vi "vector_to_xy.vi"(8 "threshold":dbl=10.0, 9 "Max Speed":dbl=3.0, 11 "Initial X, Y, BEARING":cluster{dbl, dbl, dbl}) -> (3 "Final X, Y, BEARING":cluster{dbl, dbl, dbl}={-4.992843950545212, 691.6700659397637, 27.314769230769336})   [LabVIEW 2017]
uses:
  040-typeDefs/Position.ctl
  <vilib>/myRIO/Common/Instrument Driver Framework/myRIO v1.0/Encoder/typedefs/Encoder Signal Mode.ctl
  <vilib>/myRIO/Instrument Drivers/Onboard IO/Encoder/typedefs/Encoder Reference.ctl
  <vilib>/myRIO/Common/Instrument Driver Framework/Utilities/typedefs/myRIO Generic Hardware Reference.ctl
  <vilib>/myRIO/Common/Instrument Driver Framework/Utilities/typedefs/Hardware Version Enum.ctl
  <vilib>/myRIO/Common/Instrument Driver Framework/Utilities/typedefs/myRIO v1.0 Reference.ctl
  <vilib>/myRIO/Common/Instrument Driver Framework/Utilities/typedefs/Generic FPGA Reference.ctl
  <vilib>/myRIO/Common/Instrument Driver Framework/myRIO v1.0/Encoder/typedefs/Encoder Channels Enum.ctl
  <vilib>/myRIO/Common/Instrument Driver Framework/myRIO v1.0/Encoder/typedefs/Encoder Configuration v1.0.ctl
  <vilib>/userdefined/High Color/nirio_resource_hc.ctl
  <vilib>/myRIO/Common/Instrument Driver Framework/Utilities/vis/Is FPGA Ref Available.vi
  <vilib>/myRIO/Common/Instrument Driver Framework/myRIO v1.0/Encoder/vis/myRIO v1.1 Open Encoder.vi
  <vilib>/myRIO/Instrument Drivers/Onboard IO/Encoder/vis/Read.vi
  <vilib>/myRIO/Common/Instrument Driver Framework/Utilities/vis/Validate Channels.vi
  <vilib>/myRIO/Common/Instrument Driver Framework/myRIO v1.0/Encoder/vis/myRIO v1.0 Reserve Encoder.vi
  <vilib>/myRIO/Common/Instrument Driver Framework/myRIO v1.0/Encoder/vis/myRIO v1.0 Build MUX Configuration Encoder.vi
  <vilib>/myRIO/Common/Instrument Driver Framework/myRIO v1.0/Resource Manager/vis/myRIO v1.0 Reserve Channel List.vi
  <vilib>/myRIO/Common/Instrument Driver Framework/myRIO v1.0/Resource Manager/vis/myRIO v1.0 Create Configuration List.vi
  <vilib>/myRIO/Common/Instrument Driver Framework/myRIO v1.0/Resource Manager/vis/myRIO v1.0 Reserve Channel.vi
  <vilib>/myRIO/Common/Instrument Driver Framework/myRIO v1.0/Resource Manager/vis/myRIO v1.0 Unreserve Channel.vi
  <vilib>/myRIO/Common/Instrument Driver Framework/myRIO v1.0/Resource Manager/vis/myRIO v1.0 Build Mutex Name.vi
  <vilib>/Utility/VariantDataType/GetNumericInfo.vi
  <vilib>/Utility/error.llb/Error Cluster From Error Code.vi
  <vilib>/myRIO/Common/Instrument Driver Framework/myRIO v1.0/myRIO v1.1 Open.vi
  <vilib>/myRIO/Common/Instrument Driver Framework/Utilities/vis/IO Manager.vi
  <vilib>/myRIO/Common/Instrument Driver Framework/Utilities/vis/Configuration Manager.vi
  <vilib>/myRIO/Common/Instrument Driver Framework/myRIO v1.0/Resource Manager/vis/myRIO v1.0 Configure IO.vi
  <vilib>/myRIO/Common/Instrument Driver Framework/myRIO v1.0/myRIO v1.0 Close.vi
  <vilib>/myRIO/Common/Instrument Driver Framework/myRIO v1.0/Encoder/vis/myRIO v1.0 Configure Encoder.vi
  <vilib>/myRIO/Common/Instrument Driver Framework/myRIO v1.0/Encoder/vis/myRIO v1.0 Read Encoder.vi
  <vilib>/addons/control/pid/pid.llb/PID (DBL).vi
  <vilib>/myRIO/Express VI/Onboard IO/Encoder/Encoder Express VI.xnode
  <vilib>/myRIO/Instrument Drivers/Onboard IO/Encoder/vis/myRIO Encoder Open.xnode
  <vilib>/myRIO/Common/Instrument Driver Framework/myRIO v1.0/Encoder/typedefs/Encoder Count Direction Enum.ctl
  <vilib>/addons/control/pid/NI_PID_pid.lvlib
  <vilib>/myRIO/Instrument Drivers/Onboard IO/Encoder/Encoder.lvlib
panel:
  out "X, Y, BEARING 2":cluster{dbl, dbl, dbl}={-5.221699480492852, 691.22694677004, 27.197538461538567}
  in  "Array":T1[](array[typedef])=[{"X Pos"=100.0, "Y Pos"=150.0, "Bearing"=0.0}, {"X Pos"=-100.0, "Y Pos"=300.0, "Bearing"=0.0}, {"X Pos"=100.0, "Y Pos"=450.0, "Bearing"=0.0}, {"X Pos"=0.0, "Y Pos"=600.0, "Bearing"=0.0}, {"X Pos"=0.0, "Y Pos"=700.0, "Bearing"=0.0}]
  in  "Min Speed":dbl=1.0
  out "PID Angle":cluster{"Bearing":dbl, dbl}(graph)={"Bearing"=30.937872520261912, 27.314769230769336}
  out "XY Graph":cluster{"X":dbl, "Y":dbl}[](graph)=[{"X"=-5.221699480492852, "Y"=691.22694677004}, {"X"=-4.992843950545212, "Y"=691.6700659397637}]
  in  "PID gains":T2={"proportional gain (Kc)"=0.05, "integral time (Ti, min)"=0.05, "derivative time (Td, min)"=0.0} {"derivative time (Td, min)" format="%.3f"; "integral time (Ti, min)" format="%.3f"; "proportional gain (Kc)" format="%.3f"}
  in  "stop":bool
  out "OUTPUT B":dbl(slide)=0.6 scale=-10.0..10.0
  out "OUTPUT A":dbl(slide)=1.4816000000000713 scale=-10.0..10.0
  out "PID A":T3(graph)={"Setpoint"=1.3414004312104115, "output"=0.09438687184526344, "dx/dt"=1.4816000000000713}
  out "PID B":T3(graph)={"Setpoint"=0.6585995687895885, "output"=0.05545907338162134, "dx/dt"=0.6}
  out "Setpoint A":dbl(slide)=1.3414004312104115 scale=-10.0..10.0
  out "Setpoint B":dbl(slide)=0.6585995687895885 scale=-10.0..10.0
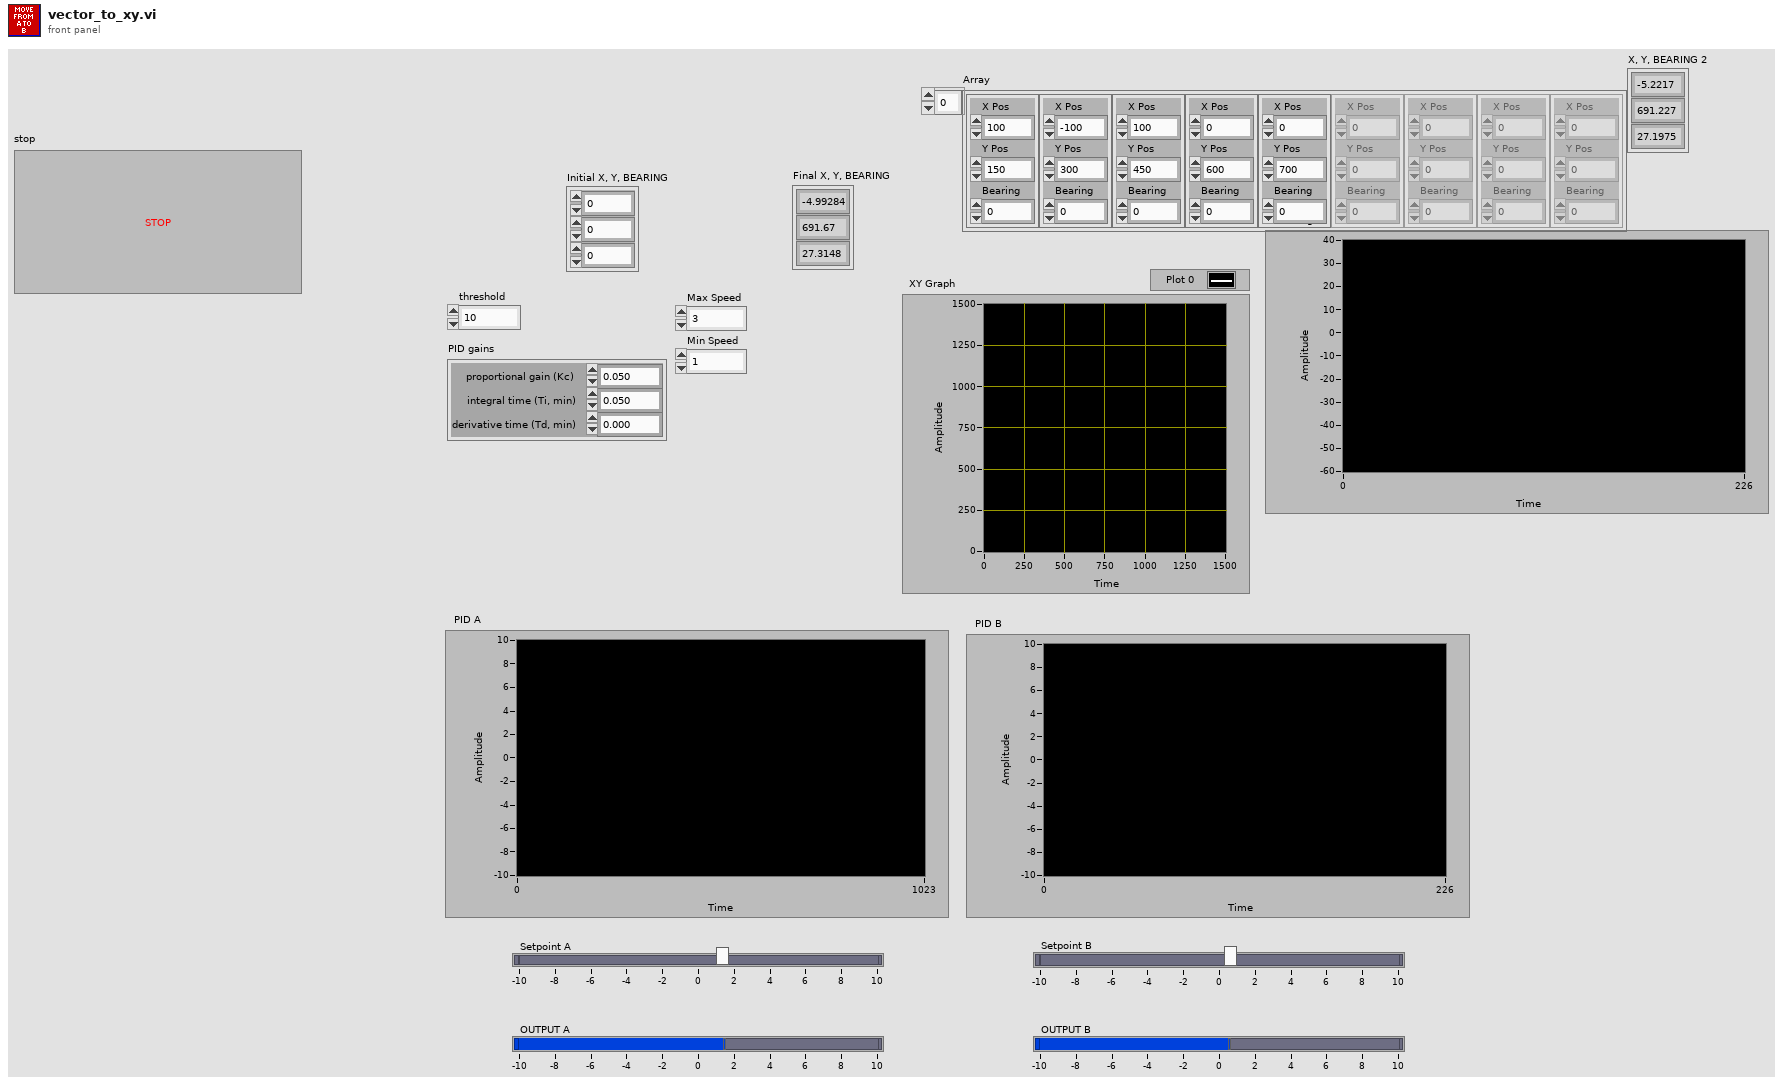
[diagram p1: front panel]
types:
  T1 = typedef "Position.ctl" = cluster{"X Pos":dbl, "Y Pos":dbl, "Bearing":dbl}
  T2 = cluster{"proportional gain (Kc)":dbl, "integral time (Ti, min)":dbl, "derivative time (Td, min)":dbl}
  T3 = cluster{"Setpoint":dbl, "output":dbl, "dx/dt":dbl}
  T4 = typedef "Encoder.lvlib/Encoder Reference.ctl" = cluster{"myRIO Reference":T5, "Encoder Channels Enum":T9}
  T5 = typedef "myRIO Generic Hardware Reference.ctl" = cluster{"myRIO Model":T6, "myRIO Hardware Reference":T7}
  T6 = typedef "Hardware Version Enum.ctl" = enum16{"Unknown", "myRIO-1900", "myRIO-1950", "roboRIO", "NI ELVIS RIO CM"}
  T7 = typedef "myRIO v1.0 Reference.ctl" = cluster{"Generic FPGA Reference":T8, "Allow multiple opens":bool}
  T8 = typedef "Generic FPGA Reference.ctl" = refnum<k20>
  T9 = typedef "Encoder Channels Enum.ctl" = enum16{"Not Connected", "C/ENC0", "C/ENC1", "A/ENC", "B/ENC", "DIO/ENC0", "DIO/ENC1", "DIO/ENC2", "DIO/ENC3", "DIO/ENC4"}
  T10 = typedef "Encoder Signal Mode.ctl" = enum16{"Quadrature phase signal", "Step and direction signal"}
  T11 = typedef "nirio_resource_hc.ctl" = tag
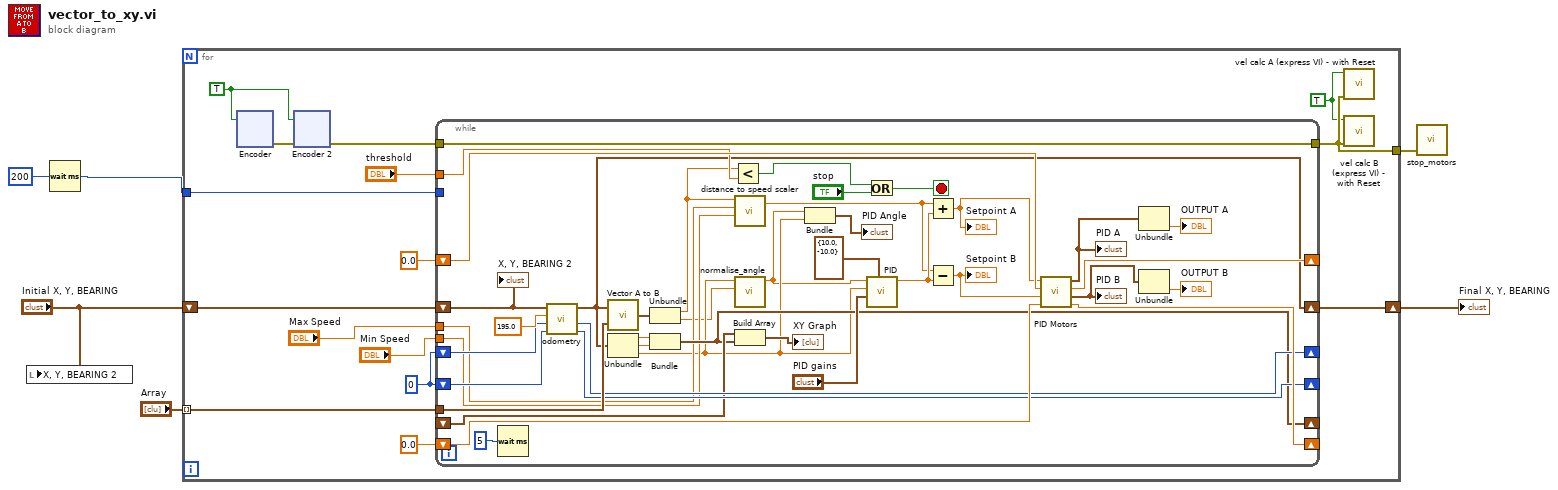
[diagram p0: block diagram]
diagram:
  n1 = local write "X, Y, BEARING 2"("Initial X, Y, BEARING") -> ()
  n2 = Wait (ms)(milliseconds to wait=u32 200) -> (millisecond timer value=w1:u32)
  n3 = for {
    shift-right: [w15] -> w6
    shift-left: "Initial X, Y, BEARING" -> [w14]
    tunnel: "Array" -> [w13] mode=indexing
    tunnel: [w9] -> w4
    tunnel: w1 -> [w7]
    w8 = TRUE ("Reinitialise")
    w11 = TRUE
    w18 = 0 ("ENCA OUT")
    n4 = xnode "Encoder"("Reset Counter"=w11) -> ("error out"=w12:errorcluster)  [unwired: 1 in, 3 out]
    n5 = xnode "Encoder 2"("error in (no error)"=w12, "Reset Counter"=w11) -> ("error out"=w10:errorcluster)  [unwired: 3 out]
    n6 = while {
      tunnel: w10 -> [w148]
      shift-right: [w150] -> _
      shift-left: 0.0 ("output A") -> [w151]
      shift-right: [w153] -> _
      shift-left: 0.0 ("output B") -> [w152]
      tunnel: [w148] -> w9
      tunnel: w13 -> [w139]
      tunnel: "threshold" -> [w135]
      shift-right: [w131] -> _
      shift-left: w18 -> [w133]
      shift-right: [w130] -> _
      shift-left: w18 -> [w132]
      shift-right: [w128] -> w15
      shift-left: w14 -> [w129]
      shift-right: [w124] -> _
      shift-left: _ -> [w125]
      tunnel: "Max Speed" -> [w119]
      tunnel: "Min Speed" -> [w118]
      tunnel: w7 -> [_]
      stop <- w136 stop-if-true
      n7 = Wait (ms)(milliseconds to wait=5 ("ENCB OUT")) -> ()  [unwired: 1 out]
      n8 = call "odometry.vi"("ENCB in"=w132, "ENCA in"=w133, "wheelbase"=195.0, "Position"=w129) -> ("ENCB OUT"=w130:i32, "ENCA OUT"=w131:i32, "X, Y, BEARING"=w128:cluster{dbl, dbl, dbl})  [unwired: 4 in]
      n9 = call "Vector A to B.vi"("Destination"=w139, "Current"=w128) -> ("vector"=w138:cluster{dbl, "Bearing":dbl})
      n10 = Unbundle(w128) -> (w126:dbl, w127:dbl, w116:dbl)
      n11 = Unbundle(w138) -> (w120:dbl, "Bearing"=w115:dbl)
      n12 = Bundle(w126, w127) -> (w124:cluster{dbl, dbl})  [unwired: 1 in]
      n13 = Less?(x=w120, y=w135) -> (x < y?=w134:bool)
      n14 = call "distance to speed scaler.vi"("Min Speed"=w118, "Max Speed"=w119, "Distance (mm)"=w120) -> ("Speed (0..10)"=w121:dbl)  [unwired: 2 in]
      n15 = call "normalise_angle.vi"("target -180 .. 180"=w115, "current"=w116) -> ("travel_direction"=w114:dbl)  [unwired: 9 in]
      n16 = Build Array(w125, w124) -> (→"XY Graph":cluster{dbl, dbl}[])
      n17 = Bundle("travel_direction"=w114, w116) -> (→"PID Angle":cluster{"travel_direction":dbl, dbl})  [unwired: 1 in]
      n18 = Or(x=w134, y="stop") -> (x .or. y?=w136:bool)
      n19 = call-poly <vilib>:"PID.vi"("output range"=cluster{"output high":dbl, "output low":dbl} {"output high"=10.0, "output low"=-10.0}, "PID gains"="PID gains", "process variable"=w116, "setpoint"=w114) -> ("output"=w143:dbl)  [unwired: 6 in, 1 out]
      n20 = Add(x=w121, y=w143) -> (x+y=w140:dbl)
      "Setpoint A" <- w140
      n21 = Subtract(x=w121, y=w143) -> (x-y=w141:dbl)
      "Setpoint B" <- w141
      n22 = call "PID Motors.vi"("input B"=w152, "Speed B"=w141, "input A"=w151, "Speed A"=w140) -> ("output B"=w153:dbl, "Speed B0"=w146:T3, "output A"=w150:dbl, "Speed A0"=w147:T3)
      "PID B" <- w146
      "PID A" <- w147
      n23 = Unbundle(w147) -> ("dx/dt"=→"OUTPUT A":dbl)  [unwired: 2 out]
      n24 = Unbundle(w146) -> ("dx/dt"=→"OUTPUT B":dbl)  [unwired: 2 out]
      "X, Y, BEARING 2" <- w129
    }
    n25 = call "vel calc A (express VI) - with Reset.vi"("error in"=w9, "Reinitialise"=w8) -> ()  [unwired: 5 in, 5 out]
    n26 = call "vel calc B (express VI) - with Reset.vi"("error in"=w9, "Reinitialise"=w8) -> ()  [unwired: 5 in, 5 out]
  }
  "Final X, Y, BEARING" <- w6
  n27 = call "stop_motors.vi"("error in (no error)"=w4) -> ()  [unwired: 4 in, 1 out]
